vi "Elevation and azimuth.vi"(2 "Antenna latitude (°)":dbl, 3 "teta (rad)":dbl, 4 "Antenna coordinates ECI":T1, 5 "Satellite coordinates ECI":T1) -> (0 "Azimuth (rad)":dbl, 1 "Elevation (rad)":dbl)   [LabVIEW 2015]
uses:
  <vilib>/Analysis/Matrix/Datatypes/RealMatrix.ctl
  <vilib>/Analysis/Matrix/NI_Matrix.lvlib
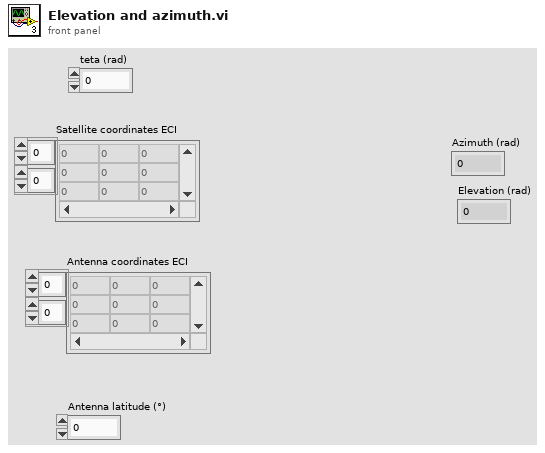
[diagram p1: front panel]
types:
  T1 = typedef "NI_Matrix.lvlib/RealMatrix.ctl" = dbl[][]
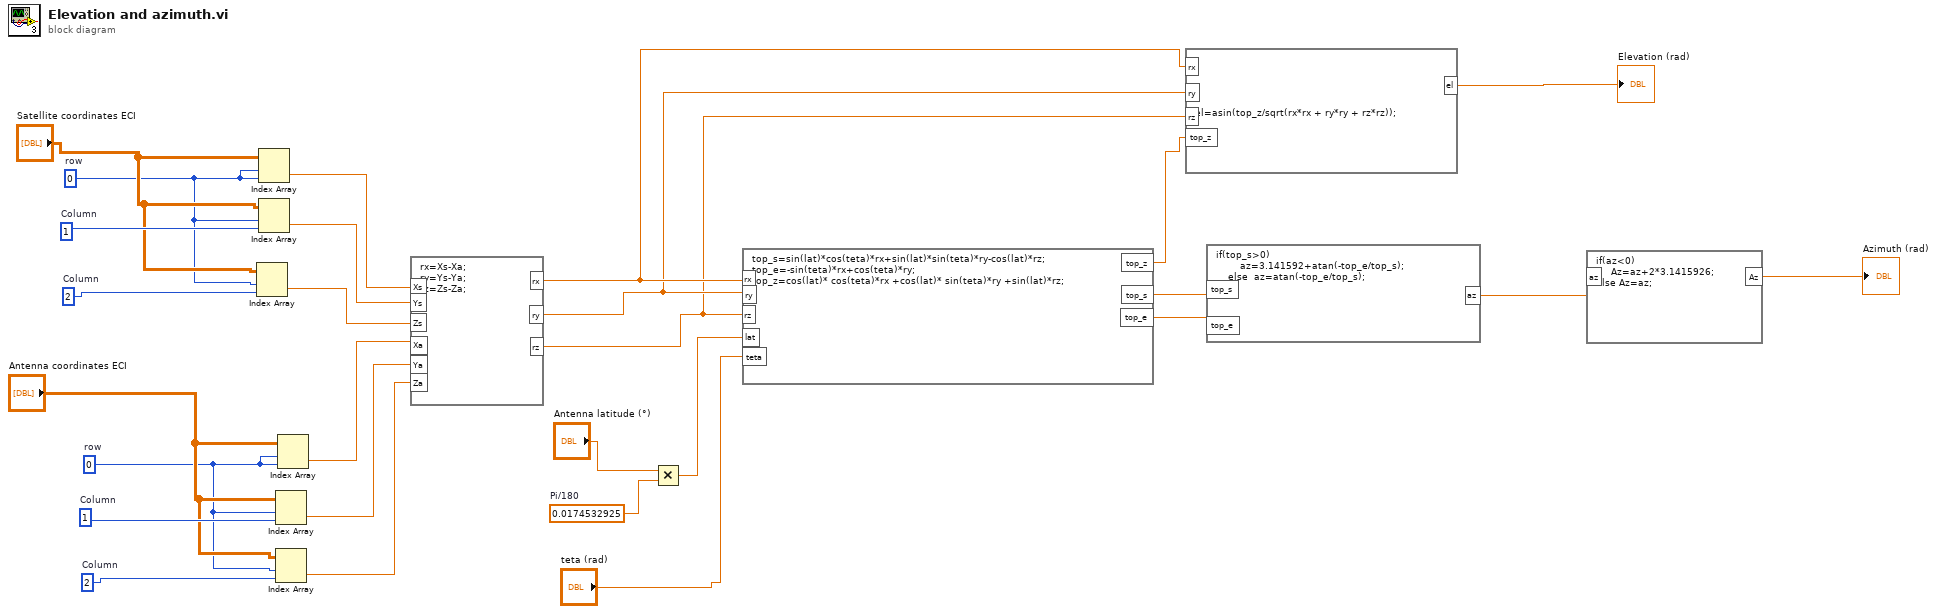
[diagram p0: block diagram]
diagram:
  w11 = 0.0174532925  # Pi/180
  w24 = 2  # Column
  w25 = 1  # Column
  w17 = 0  # row
  w26 = 2  # Column
  w27 = 1  # Column
  w18 = 0  # row
  n1 = Index Array(array="Satellite coordinates ECI", index (row)=w18, index (col)=w26) -> (element=w21:dbl)
  n2 = Index Array(array="Satellite coordinates ECI", index (row)=w18, index (col)=w18) -> (element=w19:dbl)
  n3 = Index Array(array="Satellite coordinates ECI", index (row)=w18, index (col)=w27) -> (element=w20:dbl)
  n4 = Index Array(array="Antenna coordinates ECI", index (row)=w17, index (col)=w25) -> (element=w15:dbl)
  n5 = Index Array(array="Antenna coordinates ECI", index (row)=w17, index (col)=w24) -> (element=w14:dbl)
  n6 = Index Array(array="Antenna coordinates ECI", index (row)=w17, index (col)=w17) -> (element=w16:dbl)
  n7 = formula code="rx=Xs-Xa;\nry=Ys-Ya;\nrz=Zs-Za;"("Xs"=w19, "Ys"=w20, "Zs"=w21, "Xa"=w16, "Ya"=w15, "Za"=w14) -> ("rx"=w4:dbl, "ry"=w3:dbl, "rz"=w2:dbl)
  n8 = Multiply(x="Antenna latitude (°)", y=w11) -> (x*y=w13:dbl)
  n9 = formula code="top_s=sin(lat)*cos(teta)*rx+sin(lat)*sin(teta)*ry-cos(lat)*rz;\ntop_e=-sin(teta)*rx+cos(teta)*ry;\ntop_z=cos(lat)* cos(teta)*rx +cos(lat)* sin(teta)*ry +sin(lat)*rz;"("rx"=w4, "ry"=w3, "rz"=w2, "lat"=w13, "teta"="teta (rad)") -> ("top_s"=w9:dbl, "top_e"=w8:dbl, "top_z"=w5:dbl)
  n10 = formula code="el=asin(top_z/sqrt(rx*rx + ry*ry + rz*rz));"("rx"=w4, "ry"=w3, "rz"=w2, "top_z"=w5) -> ("el"=→"Elevation (rad)":dbl)
  n11 = formula code="if(top_s>0)\n        az=3.141592+atan(-top_e/top_s);\n    else  az=atan(-top_e/top_s);"("top_s"=w9, "top_e"=w8) -> ("az"=w7:dbl)
  n12 = formula code="if(az<0)\n     Az=az+2*3.1415926;\nelse Az=az;"("az"=w7) -> ("Az"=→"Azimuth (rad)":dbl)
